vi "Predict Fiducials.vi"(11 "input cluster":T1) -> (3 "output cluster":T1)   [LabVIEW 2021, in "Component Tray.lvclass"]
uses:
  Component Tray.lvclass
  Find Component.ctl
  Controller/Camera/Machine Vision.ctl
  Controller/Camera/Camera.lvclass
panel:
  out "predicted fiducials":dbl[][](array[numeric])
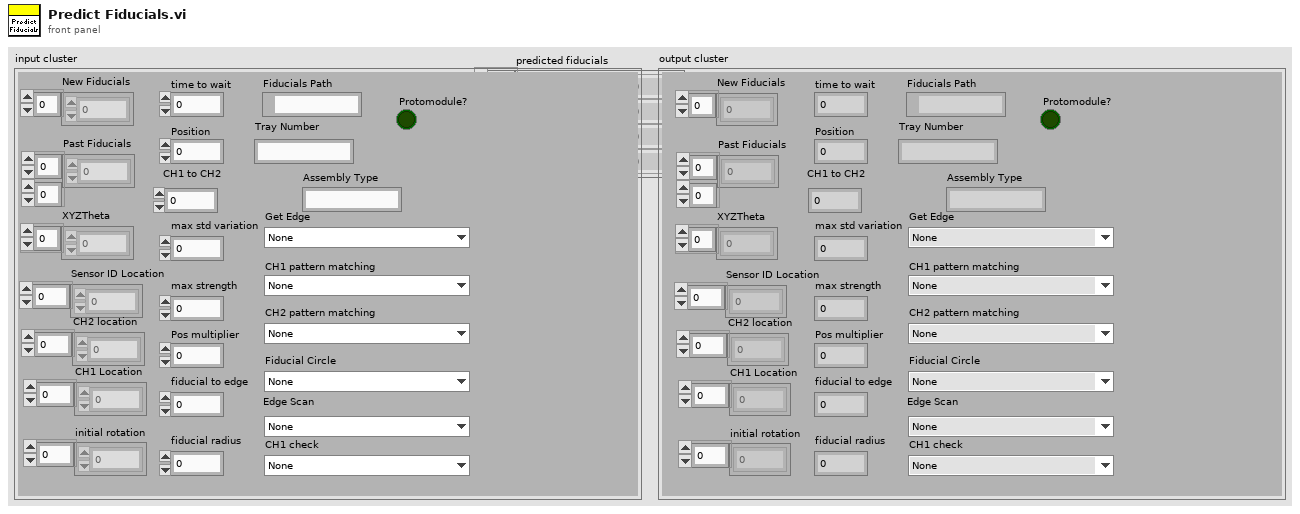
[diagram p1: front panel]
types:
  T1 = typedef "Component Tray.lvclass/Find Component.ctl" = cluster{"New Fiducials":dbl[], "Past Fiducials":dbl[][], "XYZTheta":dbl[], "Fiducials Path":path, "Position":i32, "CH1 Location":dbl[], "Sensor ID Location":dbl[], "initial rotation":dbl[], "CH2 location":dbl[], "max std variation":dbl, "max strength":dbl, "CH2 pattern matching":T2, "Fiducial Circle":T2, "Get Edge":T2, "Pos multiplier":dbl, "time to wait":u32, "fiducial to edge":dbl, "Protomodule?":bool, "Assembly Type":string, "CH1 to CH2":dbl, "Tray Number":string, "fiducial radius":dbl, "4 fiducials?":bool, "CH1 check":T2, "Edge Scan":T2, "CH1 pattern matching":T2, "Sensor Thickness":dbl}
  T2 = typedef "Camera.lvclass/Machine Vision.ctl" = enum16{"None", "Assembly Tray Circle", "Assembly Tray Fiducial", "Partial Hexaboard", "sensor edge init", "HB edge init", "sensor edge pos1", "sensor edge pos2", "HB edge pos1", "HB edge pos2", "Sensor CH1-2", "HB CH1", "HB CH2", "V3 Sensor Circle", "Hexaboard Circle", "sensor CH1 check", "HB CH1 check "}
  T3 = typedef "File Paths.ctl" = cluster{"Glue Pattern Folder":path, "Carrier Tray Folder":path, "Pick Up Tool Fixture Folder":path, "Components Folder":path, "Bellows Tool Offset.txt":path, "Pick Up Tool Offset.txt":path, "Dispense Tip Offset.txt":path, "Log Files":path, "Gantry Assembly Map.txt":path, "Syringe and offset map.txt":path, "Controllers Folder":path, "Local dbase config":path}
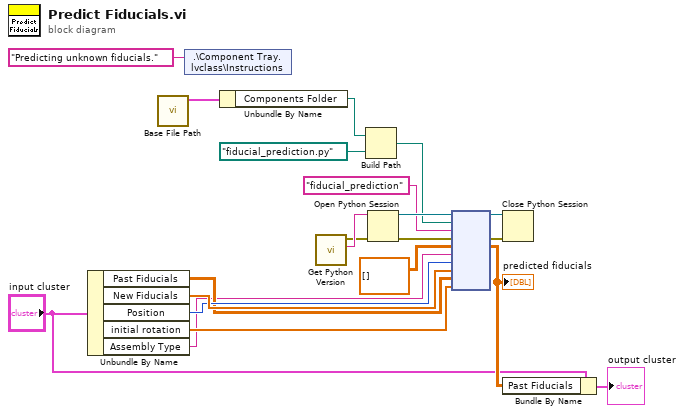
[diagram p0: block diagram]
diagram:
  n1 = Unbundle By Name("input cluster") -> ("Past Fiducials"=w19:dbl[][], "New Fiducials"=w21:dbl[], "Position"=w20:i32, "initial rotation"=w18:dbl[], "Assembly Type"=w17:string)
  n2 = call "Base File Path.vi"() -> ("Paths Out"=w16:T3)  [unwired: 11 in]
  n3 = shared-variable ".\\Component Tray.lvclass\\Instructions"("Predicting unknown fiducials." ("Instructions")) -> ()  [unwired: 1 in, 1 out]
  n4 = Unbundle By Name(w16) -> ("Components Folder"=w12:path)
  n5 = call "Get Python Version.vi"() -> ("Python Version"=w15:string, "error out"=w14:errorcluster)  [unwired: 10 in]
  n6 = Build Path(base path=w12, name or relative path=path "fiducial_prediction.py") -> (appended path=w10:path)
  n7 = Open Python Session(python version=w15, 3:w14) -> (session out=w11:refnum<k35>, error out=w8:errorcluster)  [unwired: 1 in]
  n8 = node(w11, w10, "fiducial_prediction" ("function name"), w8, dbl[][] [], w17, w20, w21, w19, w18) -> (w5:refnum<k35>, w4:errorcluster, w7:dbl[][])  [unwired: 5 in, 2 out]
  "predicted fiducials" <- w7
  n9 = Close Python Session(session in=w5, error in=w4) -> ()  [unwired: 1 out]
  n10 = Bundle By Name(cluster="input cluster", "Past Fiducials"=w7) -> (→"output cluster":T1)
